vi "Find If Constant Clicked Is Typedef.vi"(6 "error in (no error)":errorcluster, 9 "Constant In":refnum<vi>) -> (0 "error out":errorcluster, 2 "Is Typedef?":T1(ring), 3 "Constant Out":refnum<vi>, 4 "Type Definition/Class Path":string, 5 "Is Typedef/Class?":bool)   [LabVIEW 2020]
uses:
  <vilib>/Utility/Data Type/NI_Data Type.lvlib
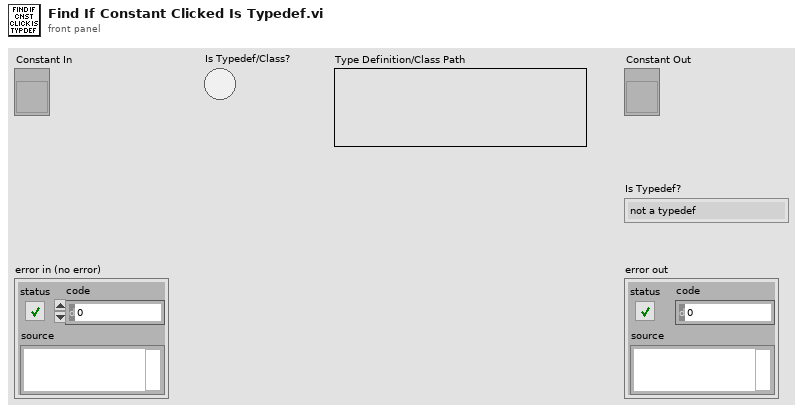
[diagram p1: front panel]
types:
  T1 = enum32{"not a typedef", "typedef", "strict typedef", "class private data"}
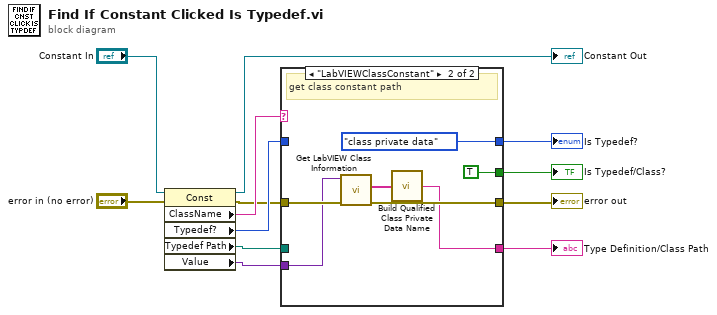
[diagram p0: block diagram]
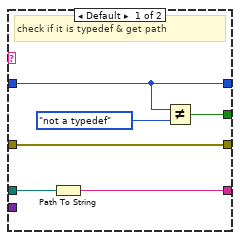
[diagram p2: hidden frame]
diagram:
  n1 = property class="Const"(reference="Constant In", error in="error in (no error)") -> (reference out=→"Constant Out":refnum<vi>, error out=w5:errorcluster, "ClassName"=w9:string, "Typedef?"=w8:T1, "Typedef Path"=w6:path, "Value"=w4:variant)
  n2 = case shown="\"LabVIEWClassConstant\"" w9 {
    tunnel: [w14 T1."class private data" ("y")] -> w7
    tunnel: w8 -> [w14 _]
    tunnel: w6 -> [w17 _]
    tunnel: w5 -> [w16 w23]
    tunnel: [w18 w20] -> w2
    tunnel: [w16 w24] -> w3
    tunnel: w4 -> [_ w22]
    tunnel: [w13 TRUE] -> w1
    frame Default {
      # "check if it is typedef & get path"
      n3 = Path To String(path=w17) -> (string=w18:string)
      n4 = Not Equal?(x=w14, y=T1."not a typedef") -> (x != y?=w13:bool)
    }
    frame "LabVIEWClassConstant" {
      # "get class constant path"
      n5 = call <vilib>:"Get LabVIEW Class Information.vi"("error in (no error)"=w23, "variant"=w22) -> ("error out"=w24:errorcluster, "qualified LabVIEW class name"=w21:string[])  [unwired: 7 in, 1 out]
      n6 = call "Build Qualified Class Private Data Name.vi"("Qualified LabVIEW Class Name"=w21) -> ("Qualified LabVIEW Class Private Data Name"=w20:string)
    }
  }
  "error out" <- w3
  "Is Typedef/Class?" <- w1
  "Type Definition/Class Path" <- w2
  "Is Typedef?" <- w7
